vi "AttackerAimGoalRole.vi"(8 "error in (no error)":errorcluster, 9 "Robot":refnum<class "Robot.lvclass">, 10 "Game in":refnum<class "Game.lvclass">, 11 "AttackerAimGoalRole in":refnum<class "AttackerAimGoalRole.lvclass">) -> (0 "error out":errorcluster, 1 "Game out":refnum<class "Game.lvclass">, 2 "Robot out":refnum<class "Robot.lvclass">, 3 "AttackerAimGoalRole out":refnum<class "AttackerAimGoalRole.lvclass">)   [LabVIEW 2023, in "AttackerAimGoalRole.lvclass"]
uses:
  AttackerAimGoalRole.lvclass
  Game_class/Game.lvclass
  Robot_class/Robot.lvclass
  Role_class/Role.lvclass/Role.ctl
  Tacticbook_class/Tacticbook.lvclass/Tacticbook.ctl
  Tacticbook_class/Read AttackerAimGoalTactic.vi
  AttackerAimGoalTactic_class/Read States.vi
  Tacticbook_class/Write AttackerAimGoalTactic.vi
  Role_class/Read Tacticbook.vi
  Role_class/Write Tacticbook.vi
  Role_class/Write tactic_index.vi
  Role_class/Read RobotRef.vi
  Tacticbook_class/Tacticbook.lvclass
  AttackerAimGoalTactic_class/AttackerAimGoalTactic.lvclass
  AttackerAimGoalRole.lvclass/AttackerAimGoalRole.ctl
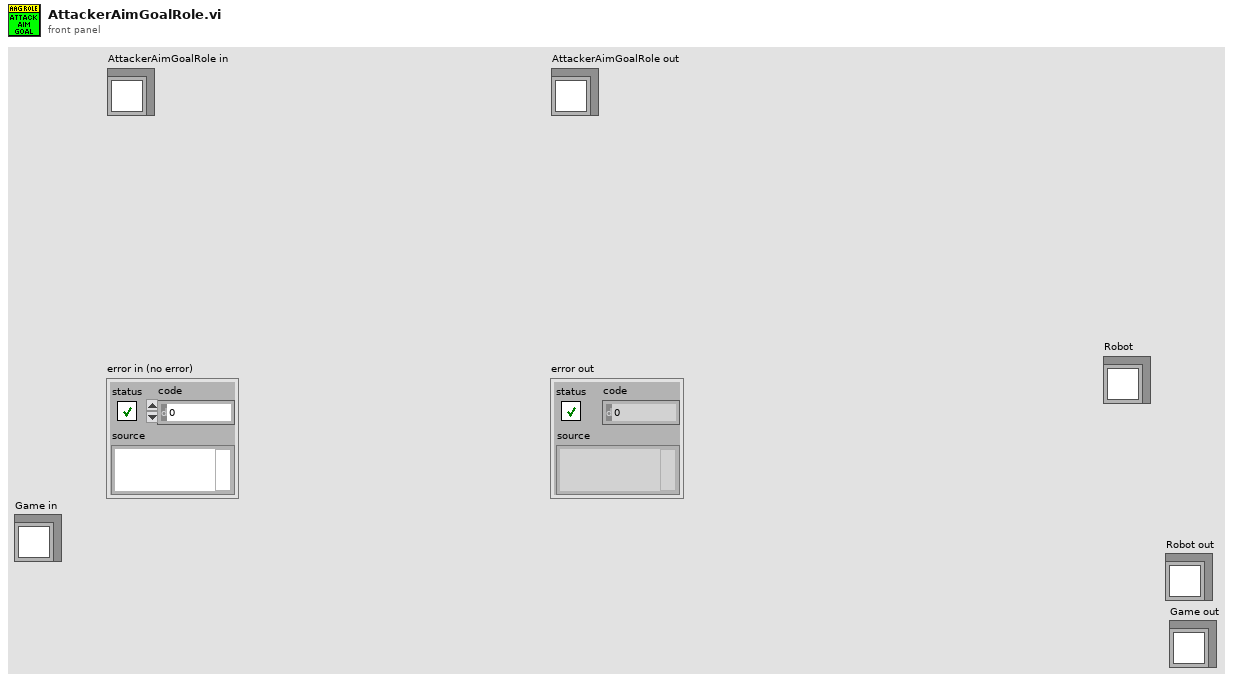
[diagram p1: front panel]
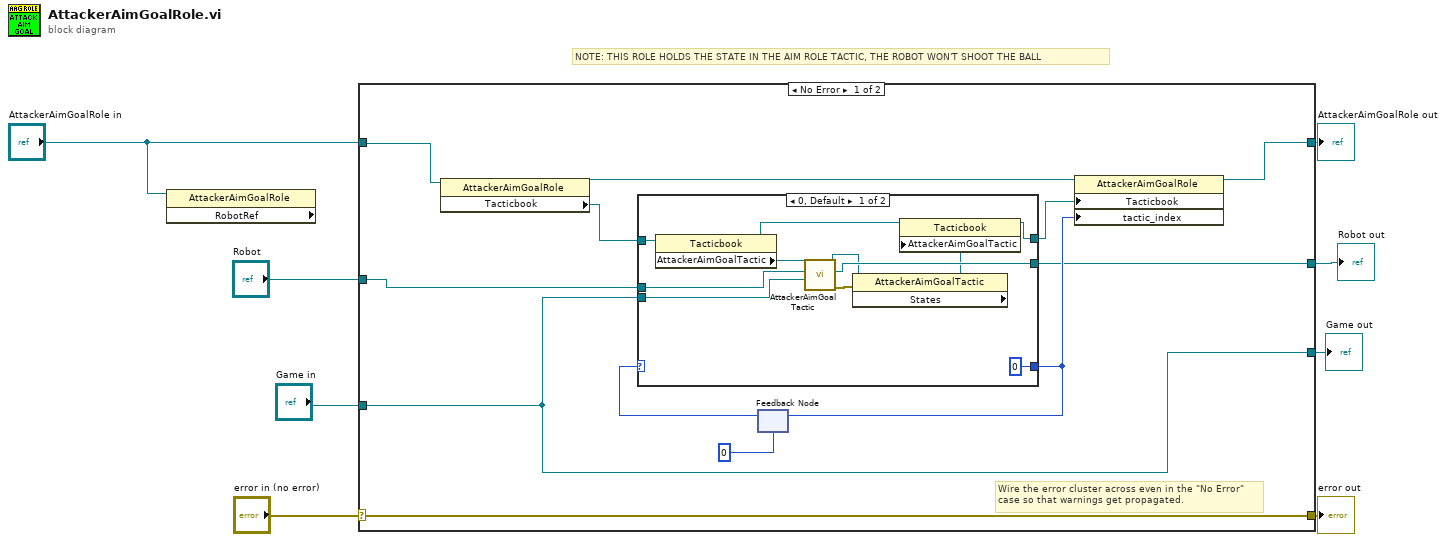
[diagram p0: block diagram]
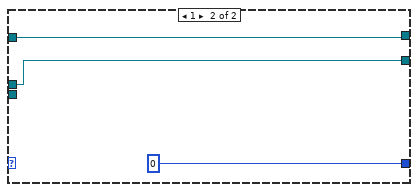
[diagram p2: hidden frame]
diagram:
  # "NOTE: THIS ROLE HOLDS THE STATE IN THE AIM ROLE TACTIC, THE ROBOT WON'T SHOOT THE BALL"
  n1 = property class="AttackerAimGoalRole" props=["RobotRef"](reference="AttackerAimGoalRole in") -> ()  [unwired: 1 in, 3 out]
  n2 = case shown="No Error" "error in (no error)" {
    selector: "error in (no error)" -> [w20 w38]
    tunnel: [w20 w38] -> w7
    tunnel: [w13 w37] -> w6
    tunnel: "AttackerAimGoalRole in" -> [w12 w37]
    tunnel: "Game in" -> [w10 w35]
    tunnel: "Robot" -> [w9 w36]
    tunnel: [w11 w36] -> w3
    tunnel: [w10 w35] -> w2
    frame No Error {
      # "Wire the error cluster across even in the \"No Error\"\ncase so that warnings get propagated."
      n3 = property class="AttackerAimGoalRole"(reference=w12) -> (reference out=w19:refnum<class "AttackerAimGoalRole.lvclass">, "Tacticbook"=w16:refnum<class "Tacticbook.lvclass">)  [unwired: 1 in, 1 out]
      n4 = feedback #1(0) -> (w17:i32)
      n5 = case shown="0, Default" w17 {
        tunnel: [0 0] -> w15
        tunnel: w16 -> [w31 w32]
        tunnel: w9 -> [w23 w34]
        tunnel: [w29 w34] -> w11
        tunnel: [w24 w32] -> w14
        tunnel: w10 -> [w21 _]
        frame 0, Default {
          n6 = property class="Tacticbook"(reference=w31) -> (reference out=w26:refnum<class "Tacticbook.lvclass">, "AttackerAimGoalTactic"=w30:refnum<class "AttackerAimGoalTactic.lvclass">)  [unwired: 1 in, 1 out]
          n7 = call-dynamic "AttackerAimGoalTactic.vi"("Game in"=w21, "Robot"=w23, "AttackerAimGoalTactic in"=w30) -> ("error out"=w28:errorcluster, "Robot out"=w29:refnum<class "Robot.lvclass">, "AttackerAimGoalTactic out"=w27:refnum<class "AttackerAimGoalTactic.lvclass">)  [unwired: 6 in]
          n8 = property class="AttackerAimGoalTactic" props=["States"](reference=w27, error in=w28) -> (reference out=w25:refnum<class "AttackerAimGoalTactic.lvclass">)  [unwired: 2 out]
          n9 = property class="Tacticbook"(reference=w26, "AttackerAimGoalTactic"=w25) -> (reference out=w24:refnum<class "Tacticbook.lvclass">)  [unwired: 1 in, 1 out]
        }
        frame 1 {
        }
      }
      n10 = feedback-in #1(w15) -> ()
      n11 = property class="AttackerAimGoalRole"(reference=w19, "Tacticbook"=w14, "tactic_index"=w15) -> (reference out=w13:refnum<class "AttackerAimGoalRole.lvclass">)  [unwired: 1 in, 1 out]
    }
    frame Error {
    }
  }
  "error out" <- w7
  "AttackerAimGoalRole out" <- w6
  "Robot out" <- w3
  "Game out" <- w2
